vi "Configure Update Rate.vi"(8 "error in (no error)":errorcluster, 10 "Update Rate (500m s)":dbl(ring)=0.5 items=["50m"=0.05, "100m"=0.1, "200m"=0.2, "500m"=0.5, "1"=1.0, "2"=2.0, "5"=5.0, "10"=10.0, "20"=20.0], 11 "VISA resource name":refnum<visa-resource-name>) -> (0 "error out":errorcluster, 3 "VISA resource name out":refnum<visa-resource-name>)   [LabVIEW 2021, in "Yokogawa WT1800 Series.lvlib"]
doc: "Configures the Data Update Interval features."
uses:
  <instrlib>/Yokogawa WT1800 Series/Yokogawa WT1800 Series.lvlib
panel:
  # "s"
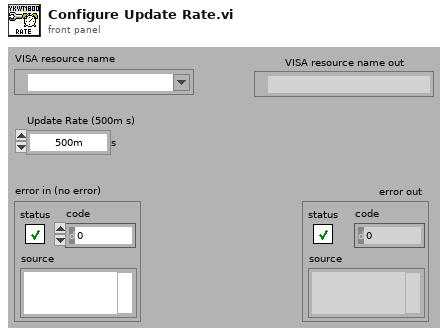
[diagram p1: front panel]
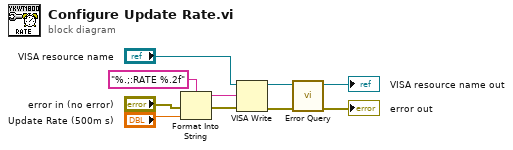
[diagram p0: block diagram]
diagram:
  n1 = Format Into String(format string="%.;:RATE %.2f" ("形式文字列"), error in="error in (no error)", "Update Rate (500m s)") -> (resulting string=w3:string, error out=w1:errorcluster)  [unwired: 1 in]
  n2 = VISA Write ("VISA書き込み")(VISA resource name="VISA resource name", write buffer=w3, error in (no error)=w1) -> (VISA resource name out=w9:refnum<visa-resource-name>, error out=w8:errorcluster)  [unwired: 1 out]
  n3 = call <instrlib>:"Error Query.vi"("error in (no error)"=w8, "VISA resource name"=w9) -> ("error out"=→"error out":errorcluster, "VISA resource name out"=→"VISA resource name out":refnum<visa-resource-name>)  [unwired: 6 in, 2 out]
